vi "Check Turret Busy (TRIAX).vi"(8 "error in (no error)":errorcluster, 11 "VISA resource name":refnum<visa-resource-name>) -> (0 "error out":errorcluster, 2 "busy?":bool, 3 "VISA resource name out":refnum<visa-resource-name>)   [LabVIEW 2009, in "JY-SPEX-TRIAX.lvlib"]
doc: "Used to poll the spectrometer after motor move or slit move commands are issued in order to see if the spectrometer is done moving."
uses:
  JY-SPEX-TRIAX.lvlib
  controls.llb/Monochromator System Number.ctl
panel:
  in  "Mono System #":T1
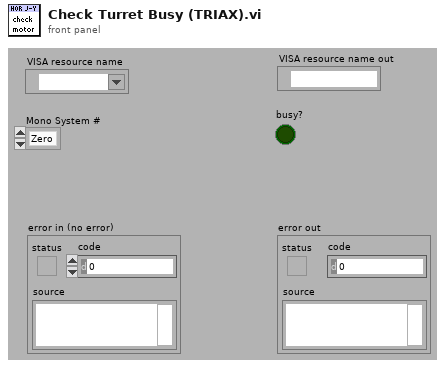
[diagram p1: front panel]
types:
  T1 = typedef "JY-SPEX-TRIAX.lvlib/Monochromator System Number.ctl" = enum16{"Zero", "One"}
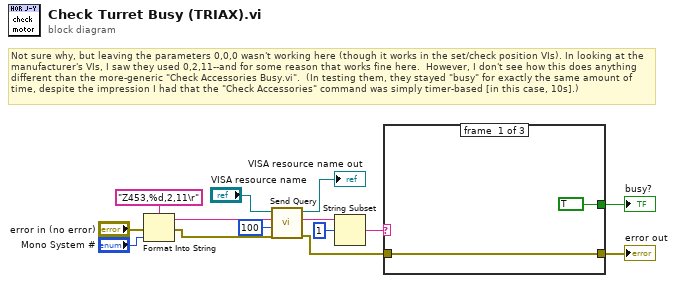
[diagram p0: block diagram]
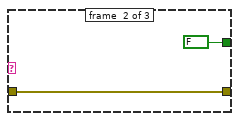
[diagram p2: hidden frame]
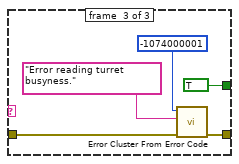
[diagram p3: hidden frame]
diagram:
  # "Not sure why, but leaving the parameters 0,0,0 wasn't working here (though it works in the set/check position VIs). In looking at the manufacturer's VIs, I saw they used 0,2,11--and for some reason that works fine here.  However, I don't see how this does anything different than the more-generic \"Check Accessories Busy.vi\".  (In testing them, they stayed \"busy\" for exactly the same amount of time, despite the impression I had that the \"Check Accessories\" command was simply timer-based [in this case, 10s].)"
  n1 = Format Into String(format string="Z453,%d,2,11\r", error in="error in (no error)", "Mono System #") -> (resulting string=w3:string, error out=w1:errorcluster)  [unwired: 1 in]
  n2 = call "Send Query.vi"("error in (no error)"=w1, "byte count"=u32 100, "write buffer"=w3, "VISA resource name"="VISA resource name") -> ("error out"=w9:errorcluster, "read buffer"=w12:string, "VISA resource name out"=→"VISA resource name out":refnum<visa-resource-name>)  [unwired: 5 out]
  n3 = String Subset(string=w12, offset (0)=1) -> (substring=w10:string)  [unwired: 1 out]
  n4 = case shown="\"z\"" w10 {
    tunnel: w9 -> [w16 w18 w20]
    tunnel: [w16 w18 w21] -> w7
    tunnel: [TRUE FALSE TRUE] -> w6
    frame #0 {
    }
    frame #1 {
    }
    frame #2 {
      n5 = call <vilib>:"Error Cluster From Error Code.vi"("error in (no error)"=w20, "error message (\"\")"="Error reading turret busyness." ("error message (\"\")"), "error code (0)"=-1074000001) -> ("error out"=w21:errorcluster)  [unwired: 1 in, 5 out]
    }
  }
  "busy?" <- w6
  "error out" <- w7
